vi "Elevator Controller.vi"(8 "error in (no error)":errorcluster, 11 "View Model":T1) -> (0 "error out":errorcluster)   [LabVIEW 2017]
doc: "Handles all Elevator operations"
uses:
  View Model/Controls/View Model.ctl
  Configuration/Controls/Config Model.ctl
  Configuration/Controls/Config Data.ctl
  Error Handler/Controls/Error Model.ctl
  Error Handler/Controls/Error Data.ctl
  Error Handler/Controls/Error Type.ctl
  View Model/Controls/Shared Model.ctl
  Controls/Elevator Model.ctl
  Controls/Elevator Location.ctl
  Controls/Elevator CMD Data.ctl
  Controls/Elevator Commands.ctl
  Controls/Elevator Overhead.ctl
  Controls/Elevator States.ctl
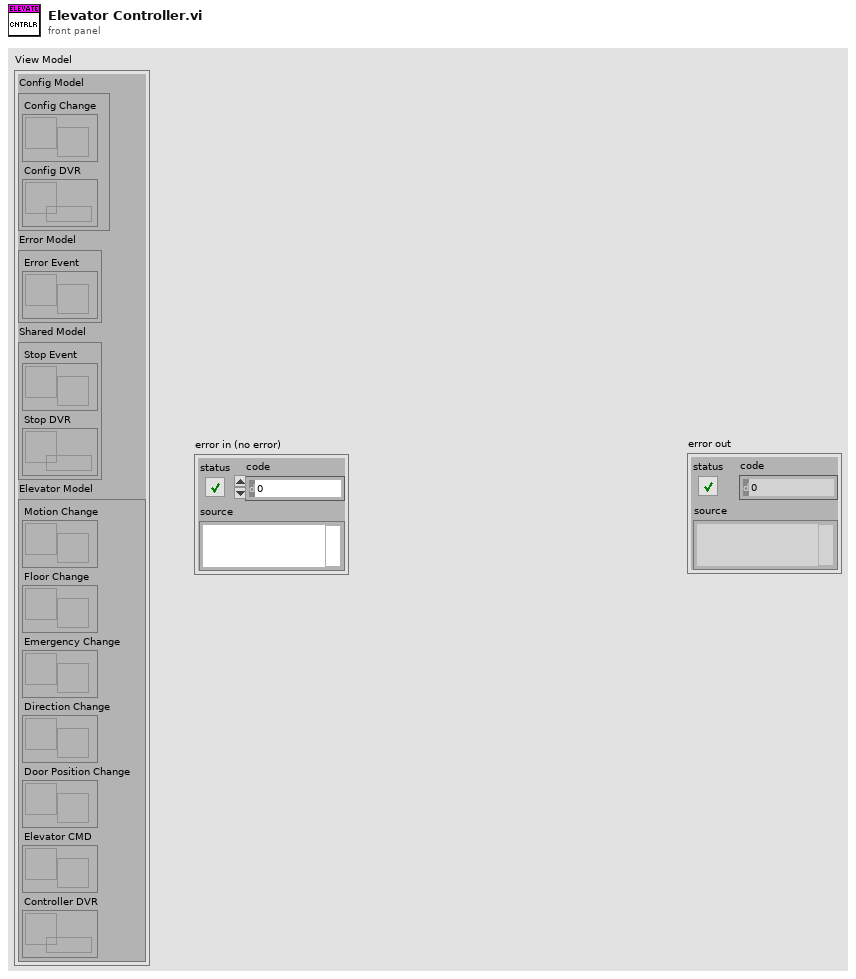
[diagram p1: front panel]
types:
  T1 = typedef "View Model.ctl" = cluster{"Config Model":T2, "Error Model":T3, "Shared Model":T4, "Elevator Model":T5}
  T2 = typedef "Config Model.ctl" = cluster{"Config Change":refnum<user-event>, "Config DVR":refnum<data-value>}
  T3 = typedef "Error Model.ctl" = cluster{"Error Event":refnum<user-event>}
  T4 = typedef "Shared Model.ctl" = cluster{"Stop Event":refnum<user-event>, "Stop DVR":refnum<data-value>}
  T5 = typedef "Elevator Model.ctl" = cluster{"Motion Change":refnum<user-event>, "Floor Change":refnum<user-event>, "Emergency Change":refnum<user-event>, "Direction Change":refnum<user-event>, "Door Position Change":refnum<user-event>, "Elevator CMD":refnum<user-event>, "Controller DVR":refnum<data-value>}
  T6 = typedef "Elevator Commands.ctl" = enum16{"Go Up", "Go Down", "Go to Floor", "Open Doors", "Close Doors", "Emergency"}
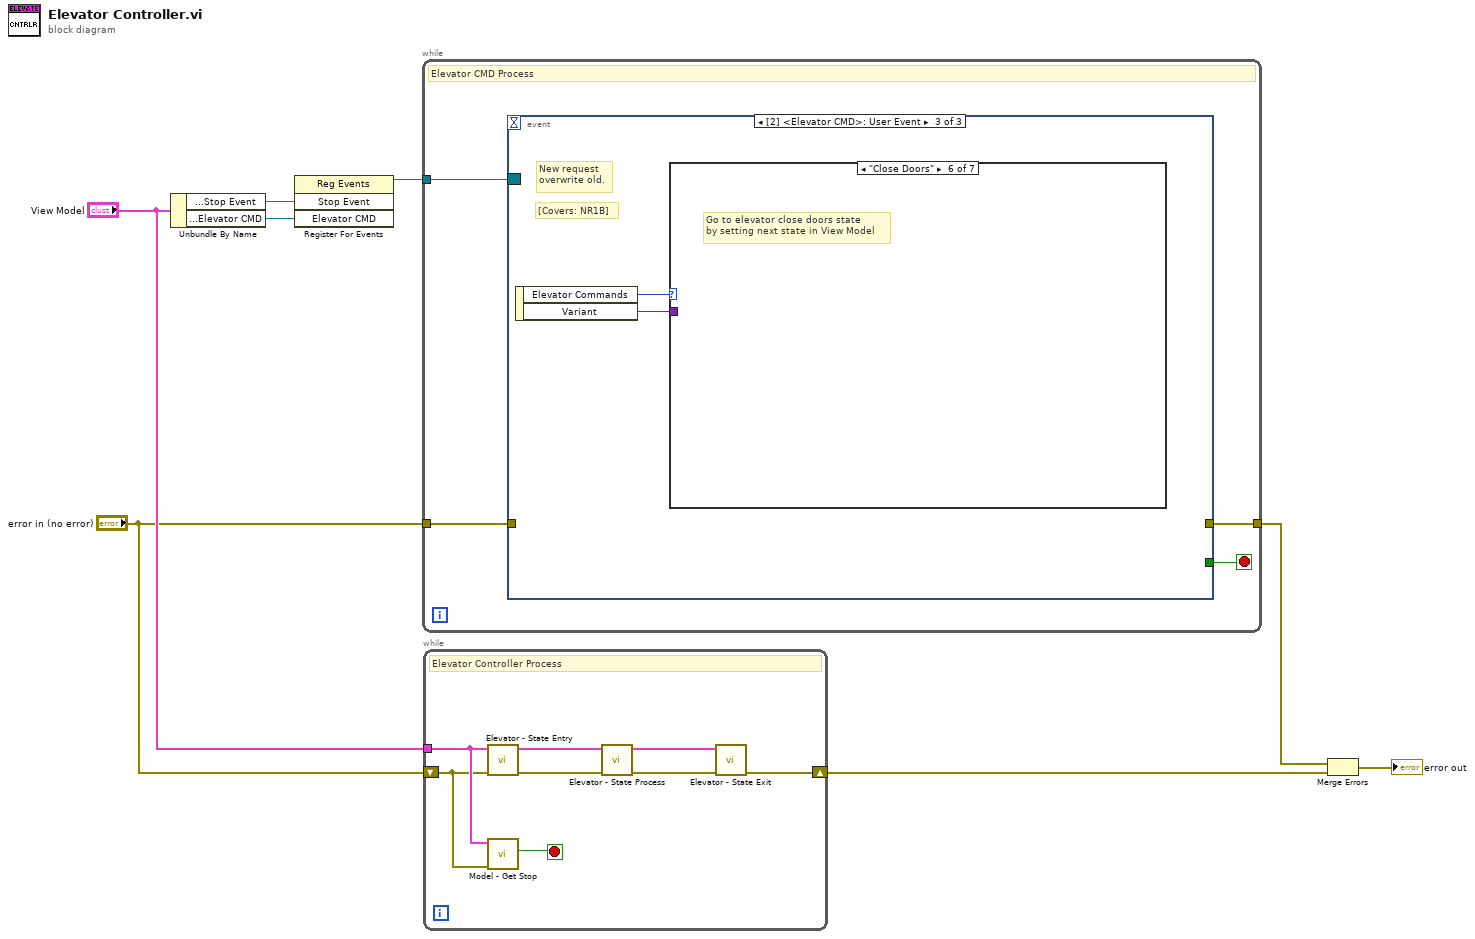
[diagram p0: block diagram]
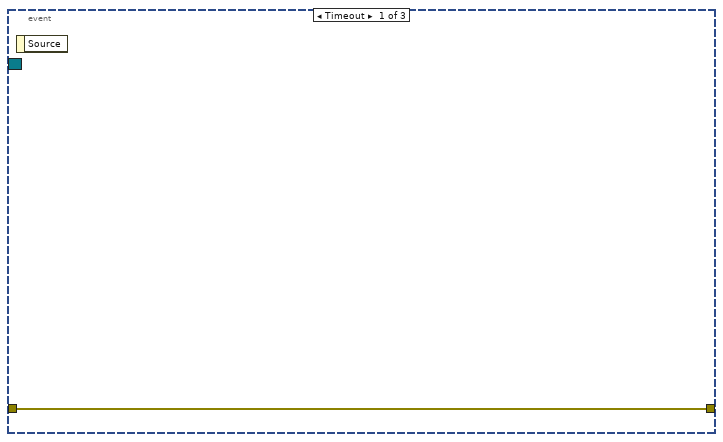
[diagram p2: hidden frame]
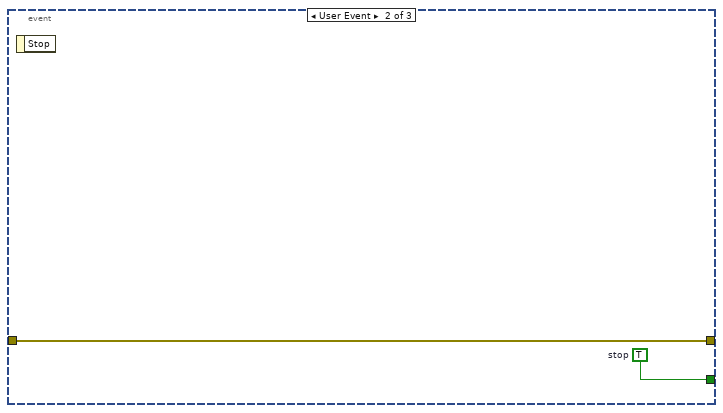
[diagram p3: hidden frame]
diagram:
  n1 = Unbundle By Name("View Model") -> ("Shared Model.Stop Event"=w8:refnum<user-event>, "Elevator Model.Elevator CMD"=w6:refnum<user-event>)
  n2 = register-events(w8, w6) -> (reference out=w7:refnum<event-registration>)  [unwired: 2 in, 1 out]
  n3 = while {
    tunnel: w7 -> [w12]
    tunnel: "error in (no error)" -> [w10]
    tunnel: [w9] -> w2
    stop <- w11 stop-if-true
    # "Elevator CMD Process"
    n4 = event shown="[2] <Elevator CMD>: User Event" {
      selector: w12 -> [_ _ _]
      dyn-events: _ -> [_ _ _]
      timeout: _ -> [_ _ _]
      tunnel: [_ w15 _] -> w11
      tunnel: w10 -> [w13 w14 _]
      tunnel: [w13 w14 _] -> w9
      event Timeout {
        n5 = event-data() -> ()  [unwired: 1 in, 1 out]
      }
      event User Event {
        w15 = TRUE  # stop
        n6 = event-data() -> ()  [unwired: 1 in, 1 out]
      }
      event User Event {
        # "[Covers: NR1B]"
        # "New request \noverwrite old."
        n7 = event-data() -> ("Elevator Commands"=w17:T6, "Variant"=w16:variant)  [unwired: 1 in]
        n8 = case shown="\"Close Doors\"" w17 {
          tunnel: w16 -> [_ _ _ _ _ _ _]
          frame Default {
          }
          frame "Go Up" {
            # "[Covers: OC3A]"
            # "Go to elevator move up state\nby setting next state in View Model"
          }
          frame "Go Down" {
            # "Go to elevator move down state\nby setting next state in View Model"
          }
          frame "Go to Floor" {
            # "[Covers: AS2B]"
            # "[Covers: AS2A]"
            # "[Covers: AS2]"
            # "#TODO\nDetermine next Elevator state - \"stop at floor\"/\"continue travel state\""
            # "[Covers: WS3]"
            # "[Covers: WS2]"
            # "#TODO\nIf elevator call requested from 1st floor, \n       then begin Open/Close Door sequence\n       else start Continue travel state"
            # "Go to elevator move up/down state\nby setting next state in View Model"
          }
          frame "Open Doors" {
            # "Go to elevator open doors state\nby setting next state in View Model"
          }
          frame "Close Doors" {
            # "Go to elevator close doors state\nby setting next state in View Model"
          }
          frame "Emergency" {
            # "Go to elevator emergency state\nby setting next state in View Model"
          }
        }
      }
    }
  }
  n9 = while {
    tunnel: "View Model" -> [w25]
    shift-right: [w21] -> w3
    shift-left: "error in (no error)" -> [w24]
    stop <- w18 stop-if-true
    # "Elevator Controller Process"
    n10 = call "Elevator - State Entry.vi"("error in (no error)"=w24, "View Model"=w25) -> ("error out"=w23:errorcluster, "View Model"=w20:T1)  [unwired: 8 in]
    n11 = call "Model - Get Stop.vi"("error in (no error)"=w24, "View Model"=w25) -> ("Stop"=w18:bool)  [unwired: 7 in, 2 out]
    n12 = call "Elevator - State Process.vi"("error in (no error)"=w23, "View Model"=w20) -> ("error out"=w22:errorcluster, "View Model"=w19:T1)  [unwired: 8 in]
    n13 = call "Elevator - State Exit.vi"("error in (no error)"=w22, "View Model"=w19) -> ("error out"=w21:errorcluster)  [unwired: 8 in, 1 out]
  }
  n14 = Merge Errors(w2, w3) -> (→"error out":errorcluster)
